vi "CheckInterface.vi"(4 "Ref 3 Active":bool, 6 "Ref 2 Active":bool, 8 "Ref 1 Active":bool, 9 "Ref 3":refnum<k21>, 10 "Ref 2":refnum<k21>, 11 "Ref 1":refnum<k21>) -> (0 "error out":errorcluster, 3 "CtrlIntf":refnum<k21>)   [LabVIEW 2020, in "FlexRay Custom Device Engine.lvlib"]
uses:
  FlexRay Custom Device Engine.lvlib
  <vilib>/Utility/error.llb/Error Cluster From Error Code.vi
  <vilib>/ErrorRing/Error Ring.xnode
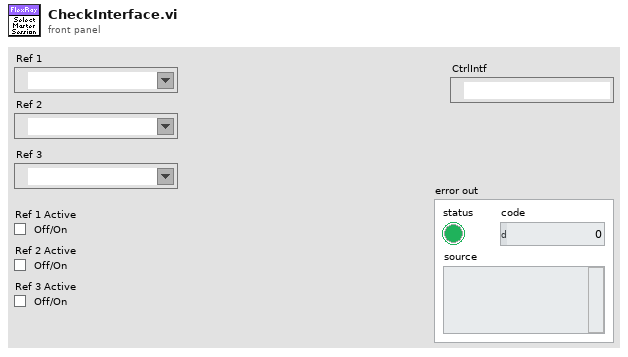
[diagram p1: front panel]
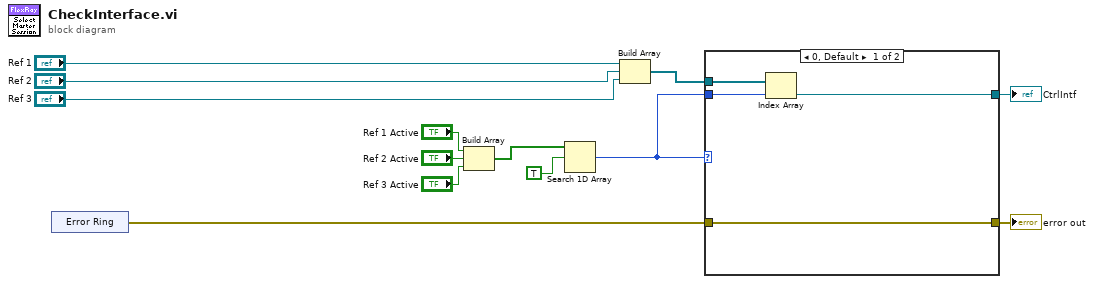
[diagram p0: block diagram]
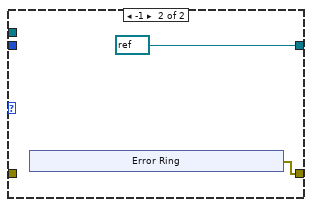
[diagram p2: hidden frame]
diagram:
  n1 = xnode "Error Ring"() -> ("error out"=w3:errorcluster)
  n2 = Build Array("Ref 1 Active", "Ref 2 Active", "Ref 3 Active") -> (w8:bool[])
  n3 = Search 1D Array(1D array=w8, element=TRUE) -> (index of element=w4:i32)  [unwired: 1 in]
  n4 = Build Array("Ref 1", "Ref 2", "Ref 3") -> (w13:refnum<k21>[])
  n5 = case shown="0, Default" w4 {
    tunnel: w4 -> [w17 _]
    tunnel: w13 -> [w16 _]
    tunnel: w3 -> [w14 _]
    tunnel: [w15 refnum<k21> refnum ("Ref 3")] -> w2
    tunnel: [w14 w18] -> w1
    frame 0, Default {
      n6 = Index Array(array=w16, index=w17) -> (element=w15:refnum<k21>)
    }
    frame -1 {
      n7 = xnode "Error Ring"() -> ("error out"=w18:errorcluster)
    }
  }
  "CtrlIntf" <- w2
  "error out" <- w1
